vi "Write Tags.vi"(8 "error in (no error)":errorcluster, 11 "State in":T1={"State"=enum."Idle", "Start Time"=timestamp(0 s since 1904-01-01), "Configuration"={"Cycle Period"=0.0, "Ismatech"={"VISA resource name"="", "Simulated?"=FALSE, "Pump Number"=1.0, "Reverse?"=FALSE}, "Masterflex"={"VISA resource name"="", "Simulated?"=FALSE, "Pump Number"=1.0, "Reverse?"=FALSE}, "Manual Entry"=0.0, "VICI Settings"={"VISA resource name"="", "Simulated?"=FALSE, "Pump Letter"="", "Reverse?"=FALSE}, "Output Device"=enum."Ismatec ISM 831C", "Tacmina Settings"={"Analog DAQ Task"="", "Digital DAQ Task"=""}, "KNF SIMDOS Settings"={"VISA resource name"="", "Simulated?"=TRUE}, "ASIA Pump C"={"ASIA Pump #"=0, "channel"=0, "Simulated"=FALSE}, "FLOM Settings"={"VISA resource name"="", "Simulated?"=TRUE, "Pump Number"=0.0}, "Pump Calibration File"=path "", "Calibration Slope"=0.0, "Calibration Y Intercept"=0.0, "Pump Cal Enum"=0, "SSI PR Settings"={"VISA resource name"="", "Simulated?"=FALSE}}, "Current Time"=timestamp(0 s since 1904-01-01), "First Iteration"=FALSE, "Data"={"Pump Speed"=0.0, "Pump Pressure"=0.0, "Pump Flow"=0.0}, "Process Name"="", "Pump On?"=enum."Off", "Output Error"=FALSE, "Log Started"=FALSE, "Overpressure Alarming"=FALSE} {"Configuration"."ASIA Pump C"."channel" min=0 max=1 step=1; "Configuration"."Masterflex"."Pump Number" min=1.0 max=20.0 step=1.0; "Configuration"."Ismatech"."Pump Number" min=1.0 max=20.0 step=1.0}) -> (0 "error out":errorcluster, 3 "State out":T1={"State"=enum."Idle", "Start Time"=timestamp(0 s since 1904-01-01), "Configuration"={"Cycle Period"=0.0, "Ismatech"={"VISA resource name"="", "Simulated?"=FALSE, "Pump Number"=1.0, "Reverse?"=FALSE}, "Masterflex"={"VISA resource name"="", "Simulated?"=FALSE, "Pump Number"=1.0, "Reverse?"=FALSE}, "Manual Entry"=0.0, "VICI Settings"={"VISA resource name"="", "Simulated?"=FALSE, "Pump Letter"="", "Reverse?"=FALSE}, "Output Device"=enum."Ismatec ISM 831C", "Tacmina Settings"={"Analog DAQ Task"="", "Digital DAQ Task"=""}, "KNF SIMDOS Settings"={"VISA resource name"="", "Simulated?"=TRUE}, "ASIA Pump C"={"ASIA Pump #"=0, "channel"=0, "Simulated"=FALSE}, "FLOM Settings"={"VISA resource name"="", "Simulated?"=TRUE, "Pump Number"=0.0}, "Pump Calibration File"=path "", "Calibration Slope"=0.0, "Calibration Y Intercept"=0.0, "Pump Cal Enum"=0, "SSI PR Settings"={"VISA resource name"="", "Simulated?"=FALSE}}, "Current Time"=timestamp(0 s since 1904-01-01), "First Iteration"=FALSE, "Data"={"Pump Speed"=0.0, "Pump Pressure"=0.0, "Pump Flow"=0.0}, "Process Name"="", "Pump On?"=enum."Off", "Output Error"=FALSE, "Log Started"=FALSE, "Overpressure Alarming"=FALSE} {"Configuration"."ASIA Pump C"."channel" min=0 max=1 step=1; "Configuration"."Masterflex"."Pump Number" min=1.0 max=20.0 step=1.0; "Configuration"."Ismatech"."Pump Number" min=1.0 max=20.0 step=1.0})   [LabVIEW 2018, in "Pump Module.lvlib" / "Pump Module Engine.lvlib"]
uses:
  Pump Module Engine.lvlib
  State Cluster.ctl
  State Enum.ctl
  Pump Module Settings Cluster.ctl
  Ismatec ISM 831C/Controls/Ismatech Settings Cluster.ctl
  Masterflex 7550-30/Controls/Settings Cluster.ctl
  VICI M50 Party Mode/Settings Cluster.ctl
  Measure Instrument/PID 2 Output Enum.ctl
  Tacmina QI/Tacmina QI DAQ Setting.ctl
  KNF Pump/Settings Cluster plus SIMDOS.ctl
  ASIA Pump/Pump Settings.ctl
  FLOM Pump/Settings Cluster.ctl
  SSI PR Class/SSI PR Settings Cluster.ctl
  Tag VIs/Tag FGV Operation Enum.ctl
  Shared Variables/Dynamic Shared Variables.lvlib
  Pump Module.lvlib
  Ismatec ISM 831C/Ismatec ISM 831C.lvlib
  Masterflex 7550-30/Masterflex 7550-30.lvlib
  Tacmina QI/Tacmina QI.lvlib
  KNF Pump/KNF SIMDOS.lvlib
  ASIA Pump.lvlib
  VICI M50 Party Mode/VICI M6 M50 Party Mode.lvlib
  FLOM Pump/FLOM Pump.lvlib
  SSI PR Class/SSI PR Pump.lvlib
panel:
  # "Output Instruments"
  # "Output Instruments"
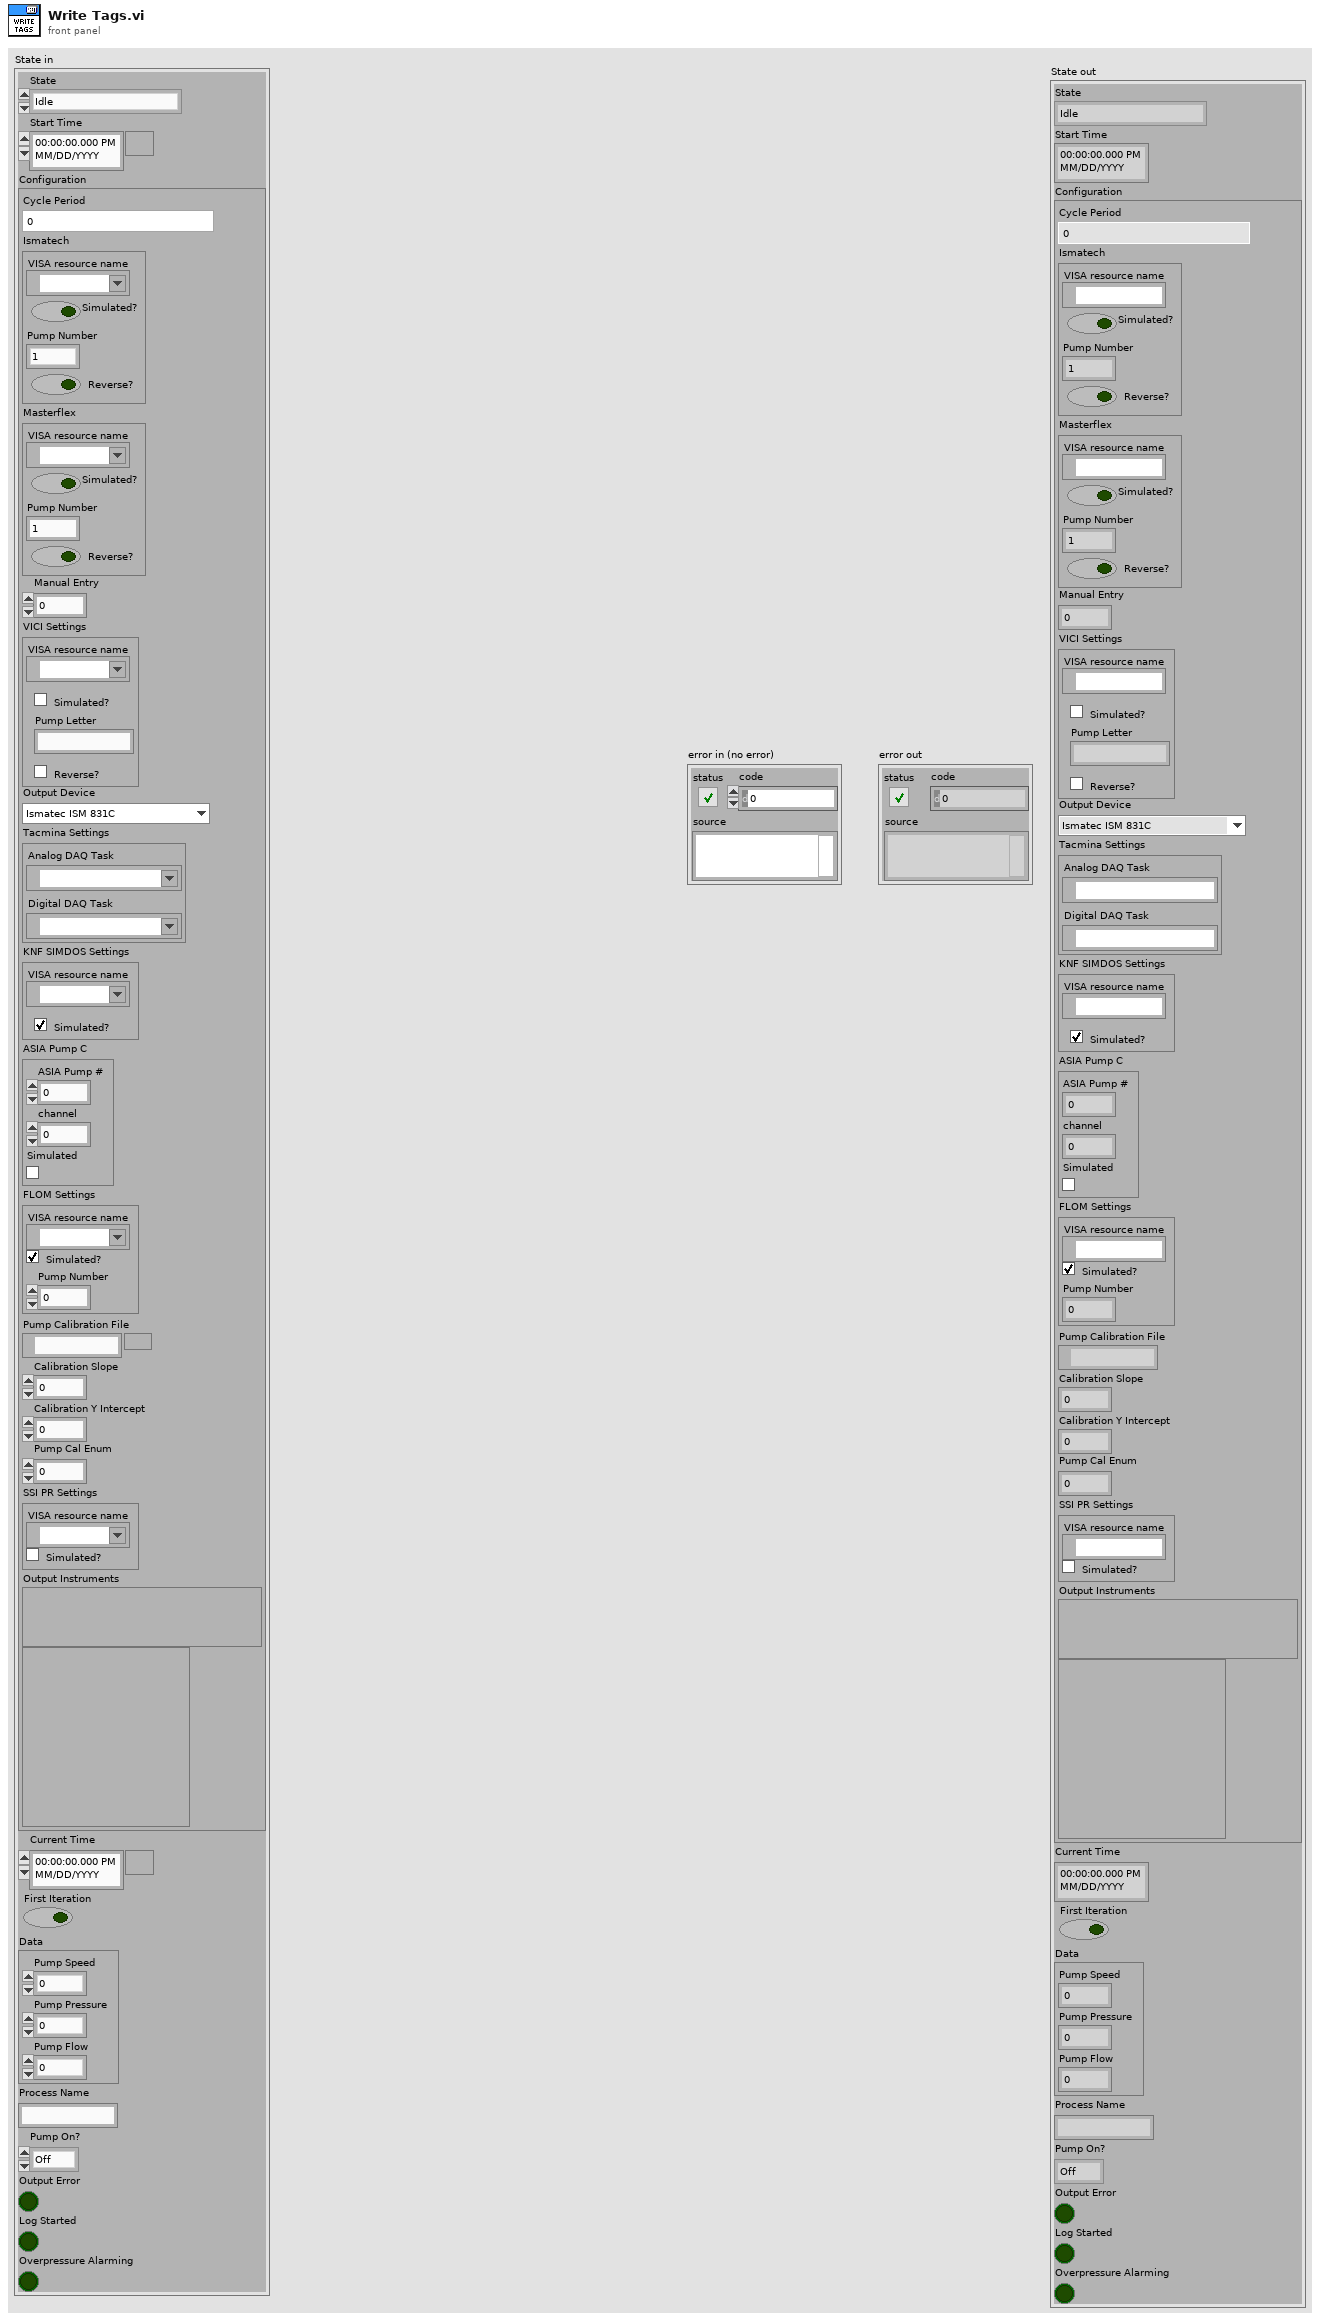
[diagram p1: front panel]
types:
  T1 = typedef "Pump Module.lvlib/Pump Module Engine.lvlib/State Cluster.ctl" = cluster{"State":T2, "Start Time":timestamp, "Configuration":T3, "Current Time":timestamp, "First Iteration":bool, "Data":cluster{"Pump Speed":dbl, "Pump Pressure":dbl, "Pump Flow":dbl}, "Process Name":string, "Pump On?":enum16{"Off", "On", "Not Initialized"}, "Output Error":bool, "Log Started":bool, "Overpressure Alarming":bool}
  T2 = typedef "Pump Module.lvlib/Pump Module Engine.lvlib/State Enum.ctl" = enum16{"Measuring", "Idle", "Paused"}
  T3 = typedef "Pump Module.lvlib/Pump Module Settings Cluster.ctl" = cluster{"Cycle Period":dbl, "Ismatech":T4, "Masterflex":T5, "Manual Entry":dbl, "VICI Settings":T6, "Output Device":T7, "Tacmina Settings":T8, "KNF SIMDOS Settings":T9, "ASIA Pump C":T10, "FLOM Settings":T11, "Pump Calibration File":path, "Calibration Slope":dbl, "Calibration Y Intercept":dbl, "Pump Cal Enum":u16, "SSI PR Settings":T12}
  T4 = typedef "Ismatec ISM 831C.lvlib/Ismatech Settings Cluster.ctl" = cluster{"VISA resource name":refnum<visa-resource-name>, "Simulated?":bool, "Pump Number":dbl, "Reverse?":bool}
  T5 = typedef "Masterflex 7550-30.lvlib/Settings Cluster.ctl" = cluster{"VISA resource name":refnum<visa-resource-name>, "Simulated?":bool, "Pump Number":dbl, "Reverse?":bool}
  T6 = typedef "VICI M6 M50 Party Mode.lvlib/Settings Cluster.ctl" = cluster{"VISA resource name":refnum<visa-resource-name>, "Simulated?":bool, "Pump Letter":string, "Reverse?":bool}
  T7 = typedef "PID 2 Output Enum.ctl" = enum16{"Default", "Ismatec ISM 831C", "Masterflex 7550-30", "VICI", "Tacmina QI", "KNF SIMDOS", "ASIA Type C", "FLOM UI-22-11", "SSI PR"}
  T8 = typedef "Tacmina QI.lvlib/Tacmina QI DAQ Setting.ctl" = cluster{"Analog DAQ Task":refnum<k21>, "Digital DAQ Task":refnum<k21>}
  T9 = typedef "KNF SIMDOS.lvlib/Settings Cluster plus SIMDOS.ctl" = cluster{"VISA resource name":refnum<visa-resource-name>, "Simulated?":bool}
  T10 = typedef "ASIA Pump.lvlib/Pump Settings.ctl" = cluster{"ASIA Pump #":i32, "channel":i32, "Simulated":bool}
  T11 = typedef "FLOM Pump.lvlib/Settings Cluster.ctl" = cluster{"VISA resource name":refnum<visa-resource-name>, "Simulated?":bool, "Pump Number":dbl}
  T12 = typedef "SSI PR Pump.lvlib/SSI PR Settings Cluster.ctl" = cluster{"VISA resource name":refnum<visa-resource-name>, "Simulated?":bool}
  T13 = typedef "Tag FGV Operation Enum.ctl" = enum16{"Init", "Set Notification Queue", "Create Tag", "Commit", "Write Tag (Numeric)", "Write Tag (Boolean)", "Read All Tags", "Read One Tag", "Delete Tag Category", "Set Alarm Parameters (Numeric)", "Set Alarm Parameters (Boolean)", "Enable All Alarms", "Disable All Alarms", "Delete All Tags", "Read Alarms", "Ack Alarm", "Read Alarm Parameters (Numeric)", "Read Alarm Parameters (Boolean)"}
  T14 = typedef "Pump Module.lvlib/Pump Module Tag Names Cluster.ctl" = cluster{"Pump Speed":string, "Pump Flow":string, "Pump Pressure":string, "Output Device Tag":string, "Overpressure Tag":string}
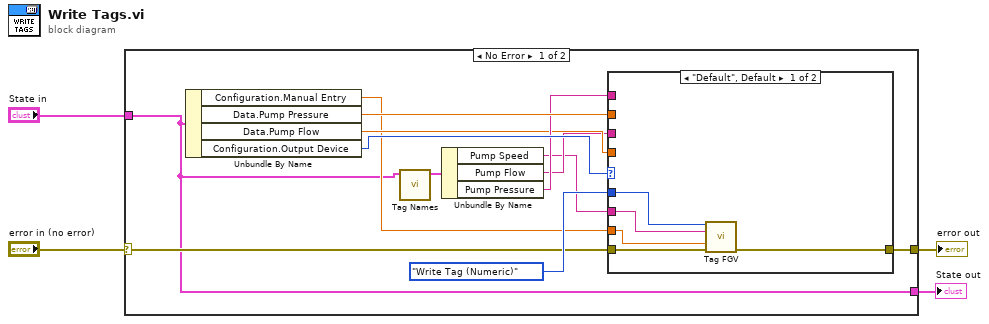
[diagram p0: block diagram]
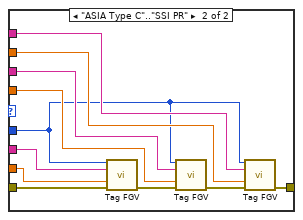
[diagram p2: hidden frame]
diagram:
  n1 = case shown="No Error" "error in (no error)" {
    selector: "error in (no error)" -> [w9 w34]
    tunnel: [w6 w34] -> w3
    tunnel: "State in" -> [w5 w33]
    tunnel: [w5 w33] -> w1
    frame No Error {
      n2 = Unbundle By Name(w5) -> ("Configuration.Manual Entry"=w8:dbl, "Data.Pump Pressure"=w14:dbl, "Data.Pump Flow"=w11:dbl, "Configuration.Output Device"=w15:T7)
      n3 = call "Tag Names.vi"("State In"=w5) -> ("Pump Module Tag Names"=w16:T14)  [unwired: 8 in, 2 out]
      n4 = Unbundle By Name(w16) -> ("Pump Speed"=w7:string, "Pump Flow"=w10:string, "Pump Pressure"=w13:string)
      n5 = case shown="\"Default\", Default" w15 {
        tunnel: w14 -> [_ w30]
        tunnel: w13 -> [_ w29]
        tunnel: Tag_FGV_Operation_Enum."Write Tag (Numeric)" ("Operation") -> [w21 w23]
        tunnel: w11 -> [_ w28]
        tunnel: w10 -> [_ w27]
        tunnel: w9 -> [w18 w26]
        tunnel: w8 -> [w19 w25]
        tunnel: w7 -> [w20 w24]
        tunnel: [w17 w22] -> w6
        frame "Default", Default {
          n6 = call "Tag FGV.vi"("Operation"=w21, "Tag Name"=w20, "Data"=w19, "error in (no error)"=w18) -> ("error out"=w17:errorcluster)  [unwired: 4 in, 7 out]
        }
        frame "ASIA Type C".."SSI PR" {
          n7 = call "Tag FGV.vi"("Operation"=w23, "Tag Name"=w24, "Data"=w25, "error in (no error)"=w26) -> ("error out"=w31:errorcluster)  [unwired: 4 in, 7 out]
          n8 = call "Tag FGV.vi"("Operation"=w23, "Tag Name"=w27, "Data"=w28, "error in (no error)"=w31) -> ("error out"=w32:errorcluster)  [unwired: 4 in, 7 out]
          n9 = call "Tag FGV.vi"("Operation"=w23, "Tag Name"=w29, "Data"=w30, "error in (no error)"=w32) -> ("error out"=w22:errorcluster)  [unwired: 4 in, 7 out]
        }
      }
    }
    frame Error {
    }
  }
  "error out" <- w3
  "State out" <- w1
